vi "Group Name Prompt.vi"(9 "Default Name (Blank)":string, 10 "Prompt":string) -> (1 "Cancelled":bool, 2 "Name":string)   [LabVIEW 2020, in "VolatusGUIElements.lvlib" / "BluelinesRedlines.lvclass"]
uses:
  BluelinesRedlines.lvclass
  BluelinesRedlines.lvclass/BluelinesRedlines.ctl
panel:
  in  "Cancel":bool
  in  "Accept":bool
  in  "Input":string
  out "Prompt Display":string
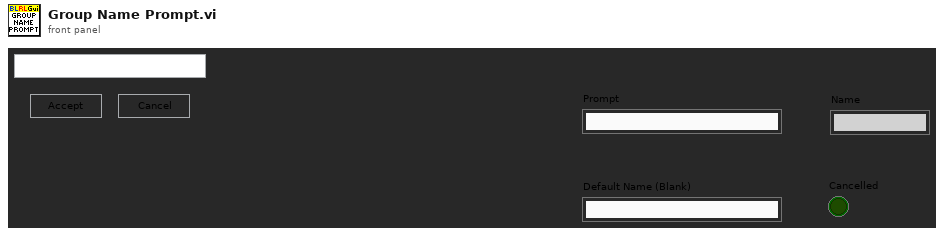
[diagram p1: front panel]
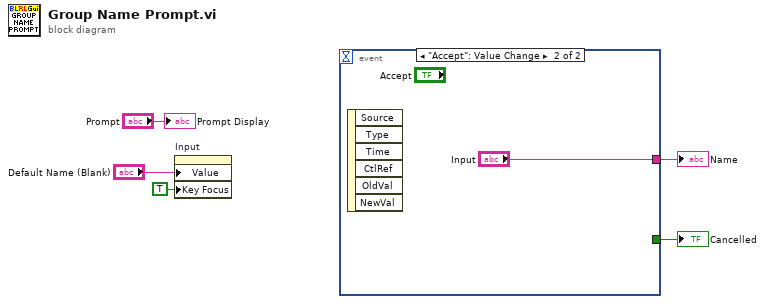
[diagram p0: block diagram]
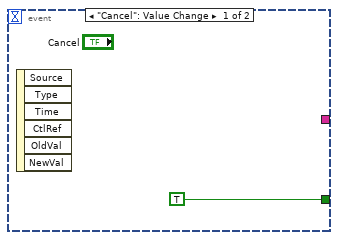
[diagram p2: hidden frame]
diagram:
  n1 = property on="Input" class="Str"("Value"="Default Name (Blank)", "Key Focus"=TRUE) -> ()  [unwired: 2 in, 2 out]
  n2 = event shown="[1] \"Accept\": Value Change" {
    selector: _ -> [_ _]
    dyn-events: _ -> [_ _]
    timeout: _ -> [_ _]
    tunnel: [TRUE _] -> w2
    tunnel: [_ "Input"] -> w1
    event "Cancel": Value Change {
      n3 = event-data() -> ()  [unwired: 1 in, 6 out]
    }
    event "Accept": Value Change {
      n4 = event-data() -> ()  [unwired: 1 in, 6 out]
    }
  }
  "Name" <- w1
  "Cancelled" <- w2
  "Prompt Display" <- "Prompt"
